vi "John_Espinoza_Lab2.vi"() -> ()   [LabVIEW 2010]
uses:
  <vilib>/Utility/file.llb/Write To Spreadsheet File (DBL).vi
  <vilib>/Analysis/NI_AALBase.lvlib
panel:
  out "?":T1(graph)
  in  "Histogram Intervals":i32
  in  "Number of Random Numbers":i32
  out "Waveform Graph\n of Random Numbers":dbl[](graph)
  in  "Desired Expected \nRandon Number":dbl
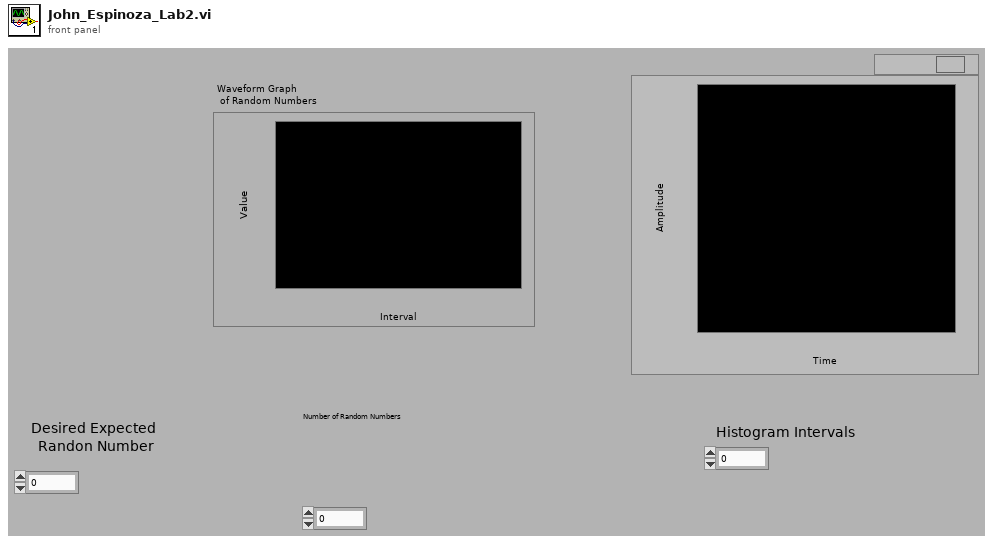
[diagram p1: front panel]
types:
  T1 = cluster{"X Values":dbl[], "Histogram: h(x)":i32[]}
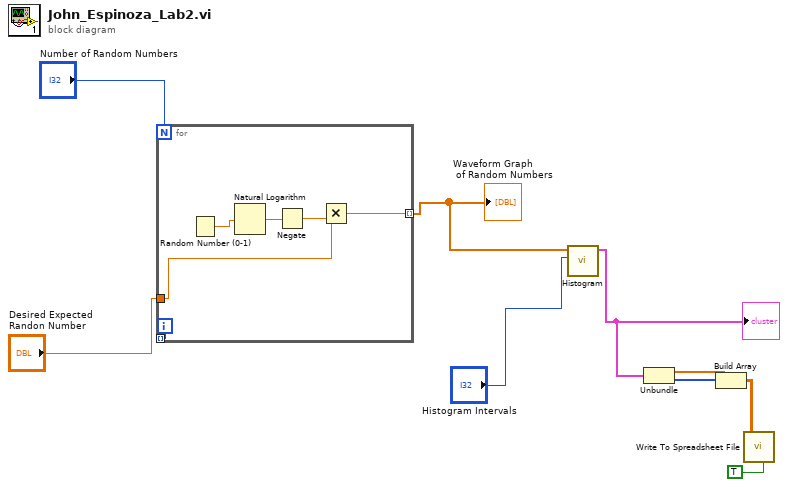
[diagram p0: block diagram]
diagram:
  n1 = for {
    N: "Number of Random Numbers" -> [_]
    tunnel: [w15] -> _ mode=indexing
    tunnel: "Desired Expected \nRandon Number" -> [w10]
    tunnel: [w11] -> w6 mode=indexing
    i -> [w15]
    n2 = Random Number (0-1)() -> (number: 0 to 1=w13:dbl)
    n3 = Natural Logarithm(1:w13) -> (0:w12:dbl)
    n4 = Negate(x=w12) -> (-x=w14:dbl)
    n5 = Multiply(x=w10, y=w14) -> (x*y=w11:dbl)
  }
  "Waveform Graph\n of Random Numbers" <- w6
  n6 = call <vilib>:"Histogram.vi"("intervals"="Histogram Intervals", "X"=w6) -> ("Histogram Graph"=w5:T1)  [unwired: 6 in, 3 out]
  "?" <- w5
  n7 = Unbundle(w5) -> ("X Values"=w4:dbl[], "Histogram: h(x)"=w3:i32[])
  n8 = Build Array(w4, w3) -> (w2:dbl[][])
  n9 = call-poly <vilib>:"Write To Spreadsheet File.vi"("transpose? (no:F)"=TRUE, "2D data"=w2) -> ()  [unwired: 6 in, 1 out]
